vi "WPI_CameraGet Image Notifier.vi"(8 "error in (no error)":errorcluster, 11 "CameraDevRef":T1) -> (0 "error out":errorcluster, 3 "Image Notifier":refnum<notifier>)   [LabVIEW 2017]
doc: "This software is licensed. Open the labview\\readme\\WPI Robotics Library Open Source License.txt file for more information."
uses:
  <vilib>/Rock Robotics/WPI/Camera/WPI_CameraDevRef.ctl
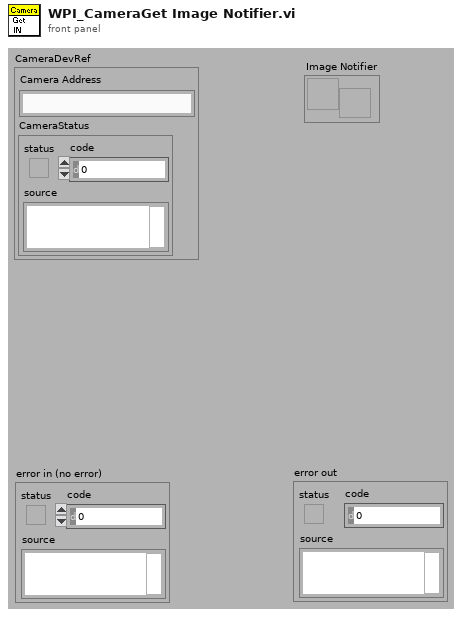
[diagram p1: front panel]
types:
  T1 = typedef "WPI_CameraDevRef.ctl" = cluster{"Camera Address":string, "CameraStatus":errorcluster}
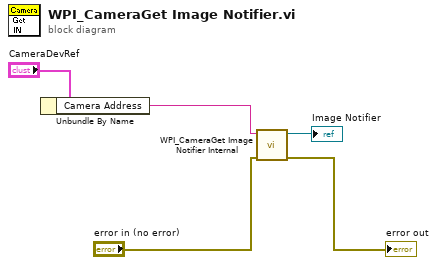
[diagram p0: block diagram]
diagram:
  n1 = Unbundle By Name("CameraDevRef") -> ("Camera Address"=w4:string)
  n2 = call <vilib>:"WPI_CameraGet Image Notifier Internal.vi"("error in (no error)"="error in (no error)", "Camera Address"=w4) -> ("error out"=→"error out":errorcluster, "Image Notifier"=→"Image Notifier":refnum<notifier>)  [unwired: 8 out]
